vi "Dashboard Main.vi"() -> ()   [LabVIEW 2016]
uses:
  <vilib>/Utility/miscctls.llb/LVRowAndColumnTypeDef.ctl
  <vilib>/event_ctls.llb/eventvkey.ctl
  <vilib>/Rock Robotics/WPI/Dashboard/WPI_DashboardLogging Global.vi
  <vilib>/Rock Robotics/Network Tables/NT Write Boolean.vi
panel:
  in  "Camera Settings Right":T1={"Frame Rate"=15, "Compression"=30, "Size"=1, "DB Camera Config"=FALSE} {"Frame Rate" scale=1.0..30.0; "Compression" scale=100.0..-1.0; "Size" items=["640x480", "320x240", "160x120"]}
  in  "Camera Name Right":string(combo)="No Camera Selection"
  out "Camera Info":cluster{"Mbps LED":bool, "Mbps":dbl, "fps":dbl} {"fps" format="%#.1g"; "Mbps" format="%#.1g"}
  in  "Camera Settings":T1={"Frame Rate"=15, "Compression"=30, "Size"=1, "DB Camera Config"=FALSE} {"Frame Rate" scale=1.0..30.0; "Compression" scale=100.0..-1.0; "Size" items=["640x480", "320x240", "160x120"]}
  in  "TCP":refnum<k5>
  in  "Rec Mode":enum32{"Stop", "Record", "Playback"}(radio)
  out "Robot IP":string
  out "Image Message":string="Timeout in Camera Communications"
  in  "Dashboard Tab":T2(tab)
  out "Pincher State":string
  out "Arm State":string
  in  "Compressor On":bool=TRUE
  in  "Battery Number":string
  in  "Match Number":u32
  out "NT Connection":bool
  out "Gyro":dbl(knob) scale=0.0..360.0
  out "Mode":T3(ring)=enum."Disconnected"
  in  "2 Gear":bool
  in  "Neutral Zone":bool
  in  "Gear Side":enum16{"Center", "Left", "Right"}(ring)
  in  "2 Gear Side":enum16{"Left", "Right"}(ring)
  in  "Alliance":enum16{"Blue", "Red"}(ring)
  in  "Routine":enum16{"Gears", "Nothing", "Reach"}(ring)
  out "Background":bool
  out "Camera Image Right":T4(plugin-control)
  in  "DB/String 9":string
  in  "DB/String 8":string
  in  "DB/String 7":string
  in  "DB/String 6":string
  in  "DB/String 5":string
  in  "DB/String 4":string
  in  "DB/String 3":string
  in  "DB/String 2":string
  in  "DB/String 1":string
  in  "DB/String 0":string
  in  "DB/Slider 0":dbl(slide) scale=0.0..5.0
  in  "DB/Slider 1":dbl(slide) scale=0.0..5.0
  in  "DB/Slider 2":dbl(slide) scale=0.0..5.0
  in  "DB/Slider 3":dbl(slide) scale=0.0..5.0
  out "DB/LED 3":bool
  out "DB/LED 2":bool
  out "DB/LED 1":bool
  out "DB/LED 0":bool
  in  "DB/Button 3":bool
  in  "DB/Button 2":bool
  in  "DB/Button 1":bool
  in  "DB/Button 0":bool caption="New Name"
  in  "Test Slider":dbl(slide) scale=0.0..100.0 scale format="%#_3g"
  in  "On/Off":bool caption="Solenoid"
  in  "Test Name":u16(ring) items=["Select the test to run..."]
  in  "Test Tree":string(tree)
  in  "Motor":cluster{"Value":dbl, "Enable":bool} {"Value" scale=-1.0..1.0 scale format="%#_3g"}
  out "Progress":T5 {"Test Progress" scale=0.0..100.0}
  in  "Rev/Fwd":cluster{"Forward":bool, "Reverse":bool}
  in  "Test Ring":u16(ring) items=["Monochrome", "Color"]
  out "Cmd Status":string
  in  "Execute Command":bool
  in  "Command Params":string[][](table)
  in  "Command Selection":i32(listbox)
  in  "CheckList":i32(listbox)
  out "Tree":string(tree)
  out "Camera Image":T4(plugin-control)
  in  "Camera Name":string(combo)="No Camera Selection"
  # "HW"
  # "HW"
  # "DO NOT PRESS SPACE OR ENTER WHILE ROBOT IS ENABLED!!!"
  # "This tab is a great place for autonomous settings and robot-specific values.\nPlace controls and indicators inside this tab and match name to\nDashboard Variables on robot. You can also delete this comment."
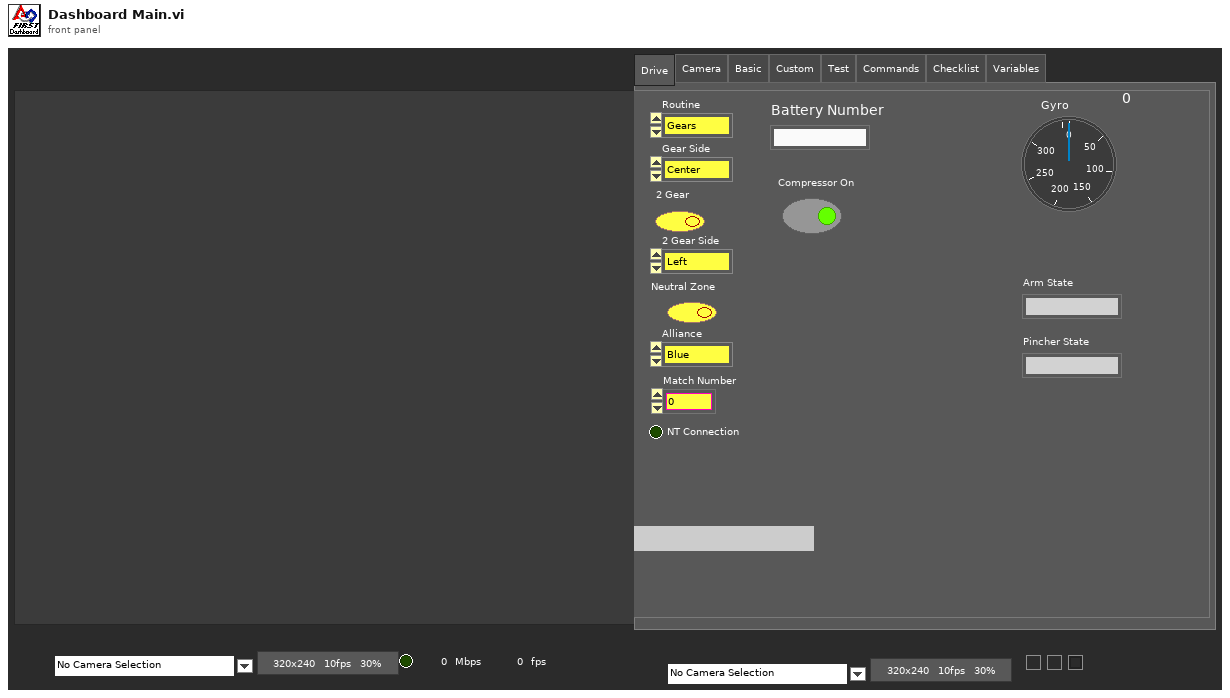
[diagram p1: front panel]
types:
  T1 = cluster{"Frame Rate":i32, "Compression":i32, "Size":u16, "DB Camera Config":bool}
  T2 = enum32{"Drive", "Camera", "Basic", "Custom", "Test", "Commands", "Checklist", "Variables"}
  T3 = enum8{"Tele-Op Disabled", "Tele-Op Enabled", "Auto Disabled", "Auto Enabled", "Test Disabled", "Test Enabled", "Disconnected", "No Code", "E-Stop"}
  T4 = typedef "IMAQ Image.ctl" = refnum<image>
  T5 = cluster{"Test Progress":u8, "Test Progress Text":string}
  T6 = cluster{"IDs":cluster{"RPC field ID":u16, "Unique ID":u16}, "String":string}
  T7 = enum32{"Drive", "Basic", "Custom", "Test", "Checklist", "Variables"}
  T8 = typedef "Image Type" = u32
  T9 = cluster{"Error Strings":string, "Disable Counts":cluster{u16, u16}, "Rail Faults":cluster{u16, u16, u16}, "Robot IP":string, "DB Mode":u8, "Event Info":cluster{"Name":string, "Type":u8, "Number":u16, "Replay":u8}}
  T10 = cluster{"Storage":cluster{"Disk Free":u64, "RAM Block":u32, "RAM free":u32}, "CPU Utilization":cluster{"CPU % ISR":sgl, "CPU % Time Crit":sgl, "CPU % Timed Str":sgl, "CPU % High":sgl, "CPU % Above":sgl, "CPU % Normal":sgl, "CPU % Low":sgl}, "CAN":cluster{"% Bus Utilization":sgl, "Bus Off Cnt":u32, "TX_FIFO Full Cnt":u32, "Receive Error Cnt":u8, "Transmit Error Cnt":u8}, "HID":cluster{"HID Outputs":u32, "Rumble Low":u16, "Rumble High":u16}[]}
  T11 = cluster{"Status bits":cluster{"Test Mode":bool, "Autonomous":bool, "Enabled":bool, "Code Start":bool, "Brownout":bool, "Reserved 2":bool, "Reserved 3":bool, "E-Stop":bool}, "Code Trace":cluster{"Disabled":bool, "TeleOp":bool, "Auto":bool, "Test":bool}, "Controller Type":enum16{"unknown", "cRIO", "roboRio"}, "Code?":enum16{"unknown", "noCode", "code"}, "Battery V":dbl}
  T12 = cluster{"Control Bits":cluster{"TestMode":bool, "Autonomous":bool, "Enabled":bool, "FMS Present":bool, bool, bool, bool, "E-Stop":bool}, "Team Station ":u8, "Countdown":sgl, "Joystick Values":cluster{"Axes":dbl[], "Buttons":bool[], "POVs":i16[]}[]}
  T13 = cluster{"Camera Image":refnum<vi>, "Dashboard Tab":refnum<vi>, "Background":refnum<vi>, "Rec Mode":refnum<vi>, "Test Slider":refnum<vi>, "On/Off ":refnum<vi>, "Test Ring":refnum<vi>, "Rev/Fwd":refnum<vi>, "Test Name":refnum<vi>, "Motor":refnum<vi>, "Progress":refnum<vi>, "CheckList":refnum<vi>, "Tree":refnum<vi>, "Test Tree":refnum<vi>, "Command Params":refnum<vi>, "Command Selection":refnum<vi>, "Execute Command":refnum<vi>, "Cmd Status":refnum<vi>, "Camera Settings":refnum<vi>, "Camera Name":refnum<vi>, "Camera Info":refnum<vi>, "Camera Settings Right":refnum<vi>, "Camera Name Right":refnum<vi>, "Camera Image Right":refnum<vi>}
  T14 = cluster{"Operation":enum16{"Update", "Clear"}, "Color Box":u32}[]
  T15 = typedef "eventvkey.ctl" = enum16{"ASCII", "Enter", "Return", "Shift", "Ctrl", "Alt", "Cmd", "Opt", "Caps", "NumLock", "Clear", "Break", "Up", "Down", "Left", "Right", "Insert", "Delete", "Home", "End", "PageUp", "PageDown", "Escape", "Help", "Pause", "ScrollLock", "F1", "F2", "F3", "F4", "F5", "F6", "F7", "F8", "F9", "F10", "F11", "F12", "F13", "F14", "F15", "F16", "F17", "F18", "F19", "F20", "F21", "F22", "F23", "F24", "Play", "VolumeUp", "VolumeDown", "Mute", "Two Byte Char"}
  T16 = cluster{"Image Size":bool, "Image Type":bool, "Pixel Value":bool, "ROI Information":bool, "Zoom Factor":bool}
  T17 = cluster{"Operation":enum16{"Update", "Clear"}, "Color Box":u32}
  T18 = typedef "LVRowAndColumnTypeDef.ctl" = cluster{"Row":i32, "Column":i32}
  T19 = cluster{"Shift":bool, "Ctrl":bool, "Alt":bool, "Cmd":bool, "Opt":bool}
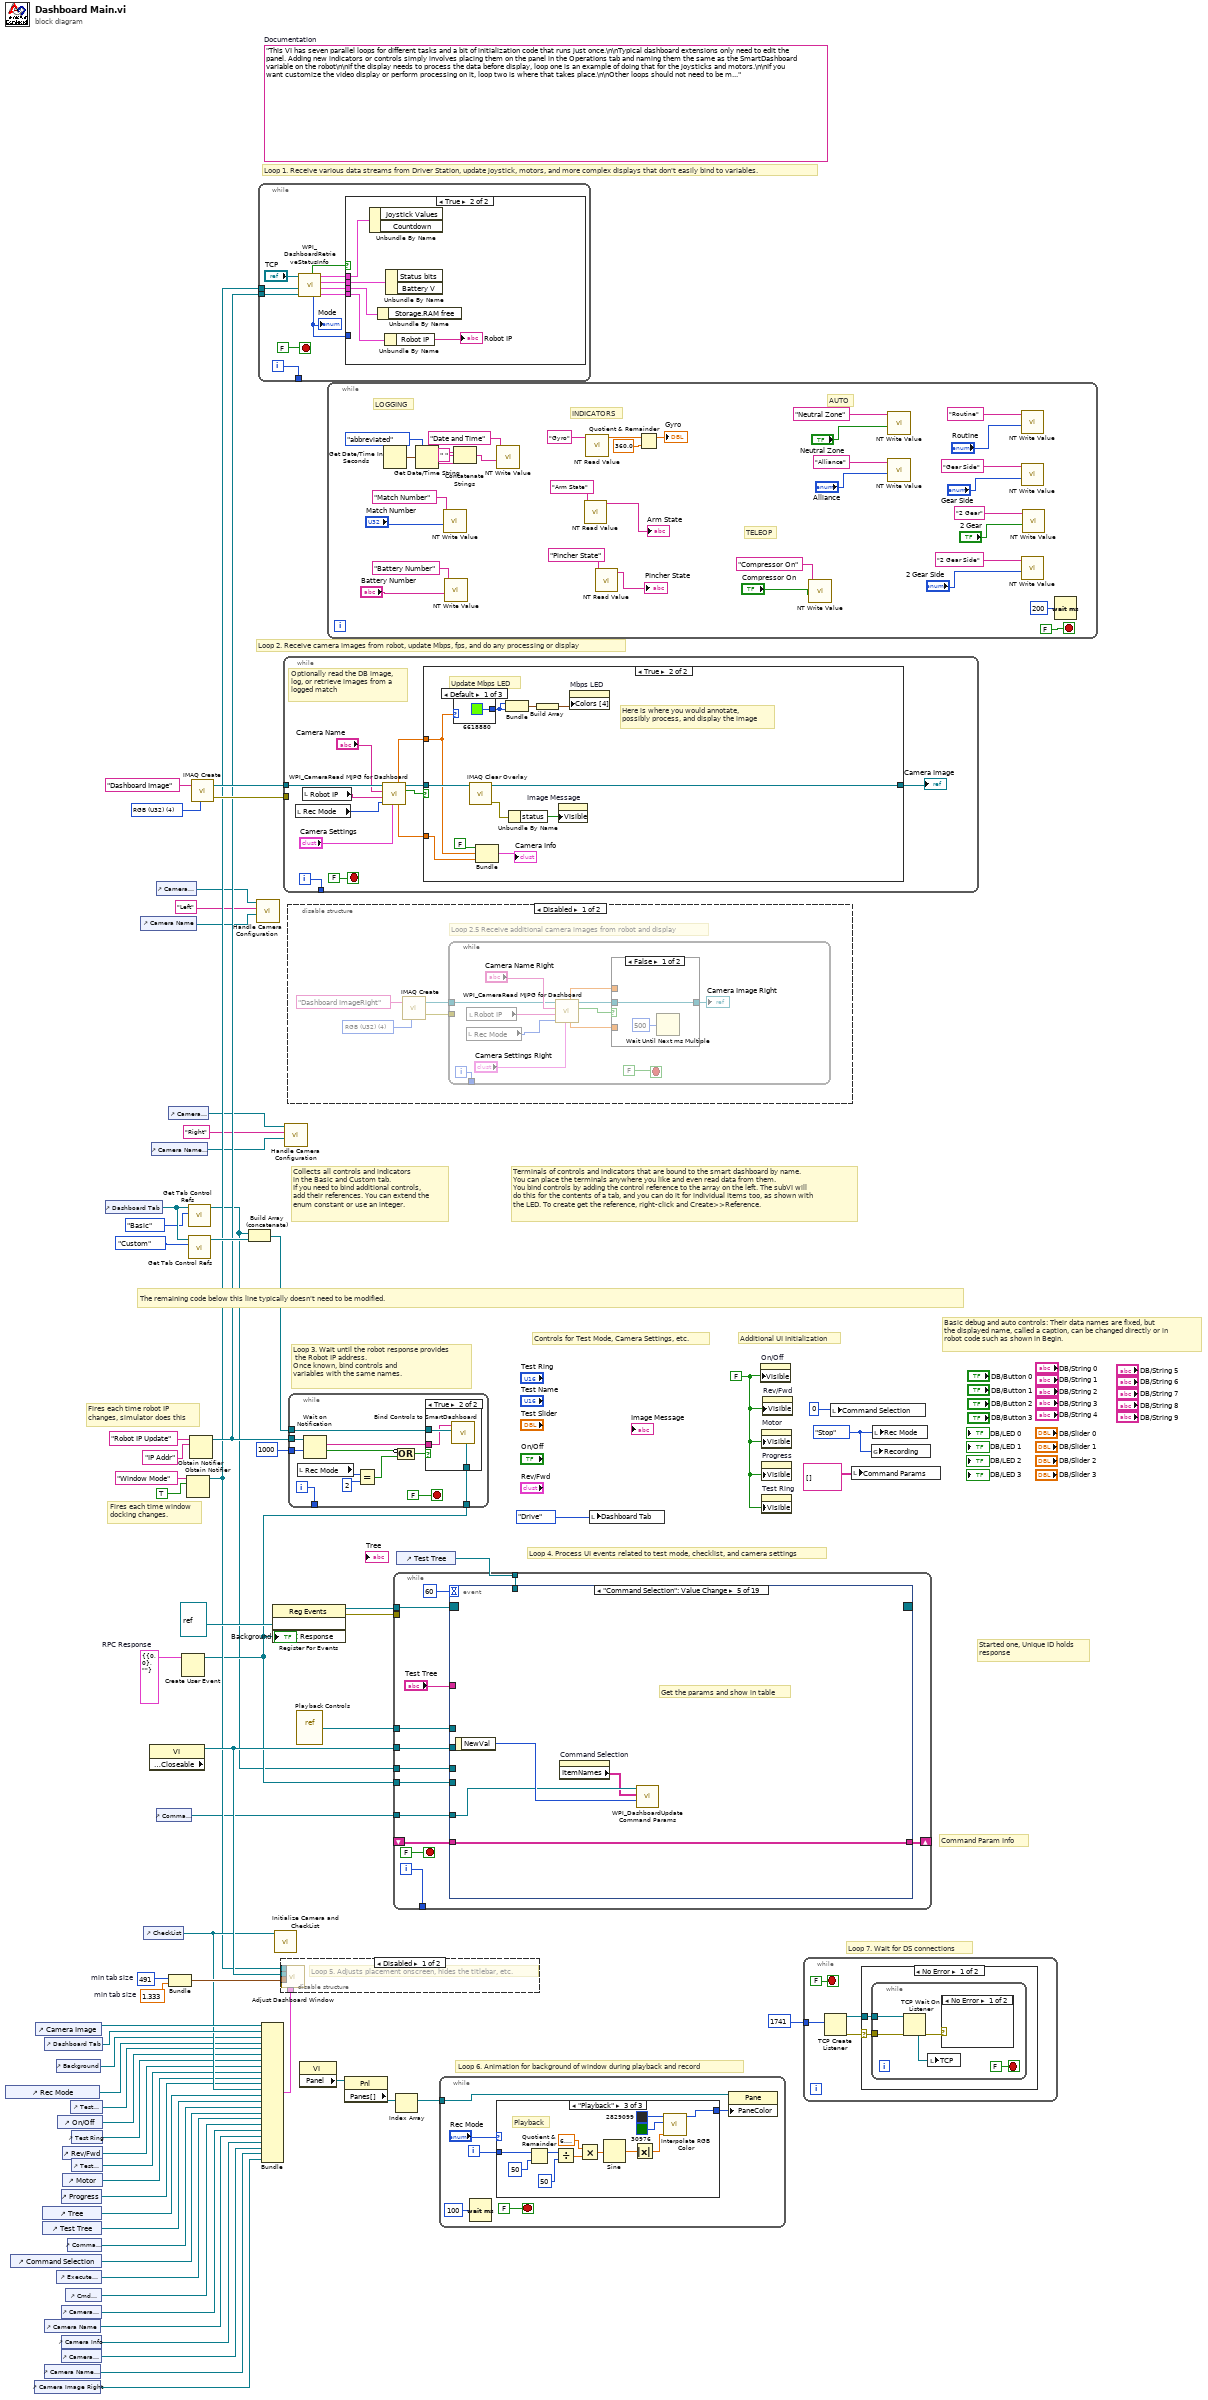
[diagram p0: block diagram]
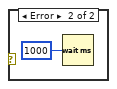
[diagram p5: hidden frame]
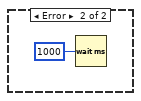
[diagram p6: hidden frame]
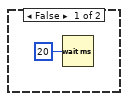
[diagram p7: hidden frame]
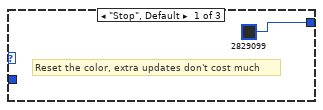
[diagram p8: hidden frame]
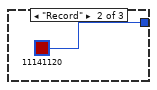
[diagram p9: hidden frame]
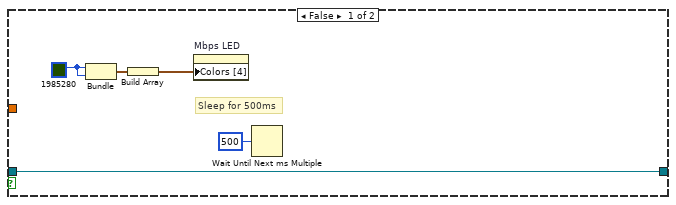
[diagram p11: hidden frame]
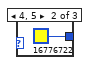
[diagram p12: hidden frame]
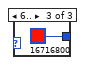
[diagram p13: hidden frame]
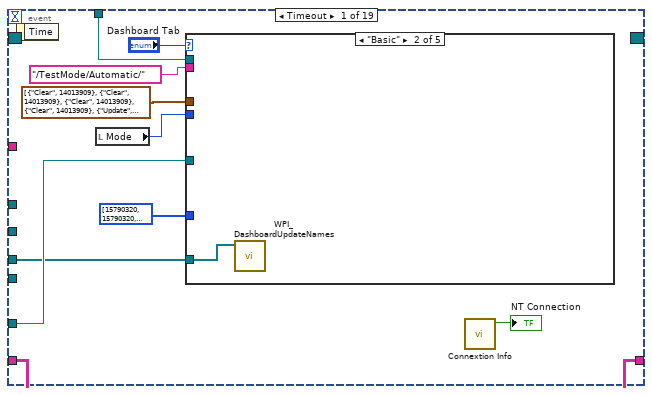
[diagram p14: hidden frame]
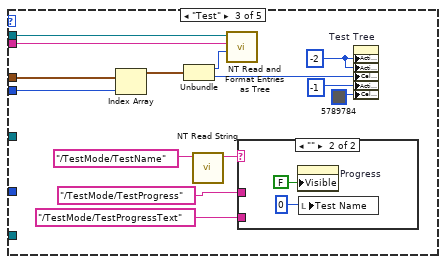
[diagram p16: hidden frame]
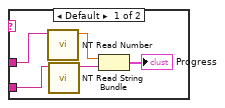
[diagram p17: hidden frame]
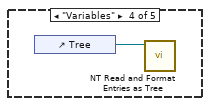
[diagram p18: hidden frame]
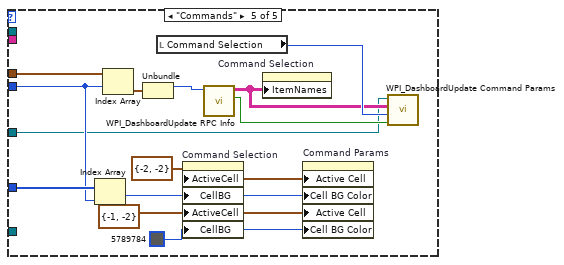
[diagram p19: hidden frame]
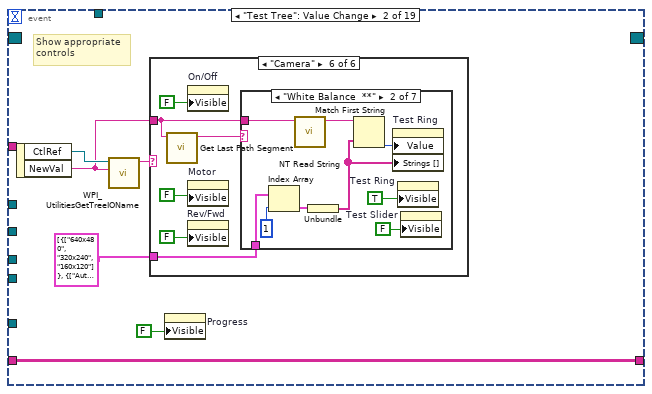
[diagram p20: hidden frame]
diagram:
  w22 = T6 {"IDs"={"RPC field ID"=0, "Unique ID"=0}, "String"=""}  # RPC Response
  w45 = 491  # min tab size
  w44 = 1.333  # min tab size
  w52 = enum32{"Stop", "Record", "Playback"}."Stop" ("Rec Mode")
  w29 = FALSE ("Visible")
  (unwired) "This VI has seven parallel loops for different tasks and a bit of initialization code that runs just once.\n\nTypical dashboard extensions only need to edit the panel. Adding new indicators or controls simply involves placing them on the panel in the Operations tab and naming them the same as the SmartDashboard variable on the robot\n\nIf the display needs to process the data before display, loop one is an example of doing that for the joysticks and motors.\n\nIf you want customize the video display or perform processing on it, loop two is where that takes place.\n\nOther loops should not need to be modified. They are pretty standard, and document the task they perform."  # Documentation
  w69 = T8 4 items=["Grayscale (U8)", "Grayscale (I16)", "Grayscale (SGL)", "Complex (CSG)", "RGB (U32)", "HSL (U32)", "RGB (U64)"] ("Image Type")
  # "Command Param Info"
  # "Started one, Unique ID holds\nresponse"
  # "Loop 7. Wait for DS connections"
  # "Basic debug and auto controls: Their data names are fixed, but\nthe displayed name, called a caption, can be changed directly or in\nrobot code such as shown in Begin."
  # "Controls for Test Mode, Camera Settings, etc."
  # "Additional UI Initialization"
  # "Loop 6. Animation for background of window during playback and record"
  # "Fires each time robot IP\nchanges, simulator does this"
  # "Fires each time window\ndocking changes."
  # "Collects all controls and indicators\nin the Basic and Custom tab.\nIf you need to bind additional controls,\nadd their references. You can extend the\nenum constant or use an integer."
  # "The remaining code below this line typically doesn't need to be modified."
  # "Loop 4. Process UI events related to test mode, checklist, and camera settings"
  # "Terminals of controls and indicators that are bound to the smart dashboard by name.\nYou can place the terminals anywhere you like and even read data from them.\nYou bind controls by adding the control reference to the array on the left. The subVI will\ndo this for the contents of a tab, and you can do it for individual items too, as shown with\nthe LED. To create get the reference, right-click and Create>>Reference."
  # "Loop 3. Wait until the robot response provides\n the Robot IP address.\nOnce known, bind controls and\nvariables with the same names."
  # "Loop 1. Receive various data streams from Driver Station, update joystick, motors, and more complex displays that don't easily bind to variables."
  # "Loop 2. Receive camera images from robot, update Mbps, fps, and do any processing or display"
  n1 = control-ref of="Rec Mode"() -> (w35:refnum<vi>)
  n2 = control-ref of="Command Selection"() -> (w21:refnum<vi>)
  n3 = control-ref of="Camera Image Right"() -> (w3:refnum<vi>)
  n4 = control-ref of="Camera Image"() -> (w47:refnum<vi>)
  n5 = control-ref of="Tree"() -> (w39:refnum<vi>)
  n6 = control-ref of="Test Tree"() -> (w38:refnum<vi>)
  n7 = control-ref of="Dashboard Tab"() -> (w46:refnum<vi>)
  n8 = control-ref of="Camera Name"() -> (w12:refnum<vi>)
  n9 = control-ref of="Camera Name Right"() -> (w4:refnum<vi>)
  n10 = control-ref of="Background"() -> (w2:refnum<vi>)
  n11 = control-ref of="Execute Command"() -> (w23:refnum<vi>)
  n12 = control-ref of="On/Off"() -> (w33:refnum<vi>)
  n13 = control-ref of="Progress"() -> (w30:refnum<vi>)
  n14 = control-ref of="Camera Settings"() -> (w13:refnum<vi>)
  n15 = control-ref of="Camera Info"() -> (w11:refnum<vi>)
  n16 = control-ref of="Camera Settings Right"() -> (w5:refnum<vi>)
  n17 = control-ref of="Rev/Fwd"() -> (w31:refnum<vi>)
  n18 = control-ref of="Motor"() -> (w36:refnum<vi>)
  n19 = control-ref of="Cmd Status"() -> (w17:refnum<vi>)
  n20 = control-ref of="Command Params"() -> (w24:refnum<vi>)
  n21 = control-ref of="Test Slider"() -> (w34:refnum<vi>)
  n22 = control-ref of="Test Ring"() -> (w32:refnum<vi>)
  n23 = control-ref of="Test Name"() -> (w37:refnum<vi>)
  n24 = control-ref of="Dashboard Tab"() -> (w50:refnum<vi>)
  n25 = control-ref of="Camera Name"() -> (w14:refnum<vi>)
  n26 = control-ref of="CheckList"() -> (w40:refnum<vi>)
  n27 = property class="VI" props=["Front Panel.Closeable"]() -> (reference out=w51:refnum<vi>)  [unwired: 2 in, 2 out]
  n28 = control-ref of="Camera Name Right"() -> (w8:refnum<vi>)
  n29 = control-ref of="Camera Settings"() -> (w15:refnum<vi>)
  n30 = control-ref of="Command Params"() -> (w16:refnum<vi>)
  n31 = control-ref of="Camera Settings Right"() -> (w9:refnum<vi>)
  n32 = Bundle("min tab size"=w45, "min tab size"=w44) -> (w43:cluster{"min tab size":i32, "min tab size":dbl})  [unwired: 1 in]
  n33 = Create User Event(user event datatype=w22) -> (user event=w18:refnum<user-event>)  [unwired: 1 in, 1 out]
  n34 = Obtain Notifier(name (unnamed)="Window Mode", notification data type=TRUE) -> (notifier out=w27:refnum<notifier>)  [unwired: 2 in, 2 out]
  n35 = call <vilib>:"Get Tab Control Refs.vi"("Page Index"=T7."Basic" ("Dashboard Tab"), "TabControl in"=w50) -> ("ControlsOnPage"=w10:refnum<vi>[])  [unwired: 9 in]
  n36 = call <vilib>:"Get Tab Control Refs.vi"("Page Index"=T7."Custom" ("Dashboard Tab"), "TabControl in"=w50) -> ("ControlsOnPage"=w49:refnum<vi>[])  [unwired: 9 in]
  n37 = Obtain Notifier(name (unnamed)="Robot IP Update", notification data type="IP Addr" ("name (unnamed)")) -> (notifier out=w28:refnum<notifier>)  [unwired: 2 in, 2 out]
  n38 = call "IMAQ Create"("Image Name"="Dashboard Image", "Image Type"=w69) -> ("New Image"=w67:T4, "error out"=w66:errorcluster)  [unwired: 2 in, 1 out]
  n39 = Build Array (concatenate)(w10, w49) -> (w48:refnum<vi>[])
  n40 = call "Handle Camera Configuration.vi"("CameraNameRef"=w14, "Camera File Name"="Left", "ClusterRef"=w15) -> ()  [unwired: 9 in]
  n41 = while {
    tunnel: w28 -> [w74]
    tunnel: w27 -> [w71]
    tunnel: [w70] -> _
    i -> [w70]
    stop <- FALSE stop-if-true
    n42 = call <vilib>:"WPI_DashboardRetrieveStatusInfo.vi"("Binding Refnum"=w74, "Window Mode Notifier"=w71, "TCP Cnx"="TCP") -> ("Power and Errors"=w75:T9, "Robot Metrics"=w78:T10, "Status Info"=w79:T11, "Control Info"=w76:T12, "Robot Mode"=w73:T3, "Process?"=w77:bool)  [unwired: 3 in]
    "Mode" <- w73
    n43 = case shown="True" w77 {
      tunnel: w79 -> [_ w86]
      tunnel: w78 -> [_ w85]
      tunnel: w76 -> [_ w84]
      tunnel: w75 -> [_ w83]
      tunnel: w73 -> [_ _]
      frame False {
        n44 = Wait (ms)(milliseconds to wait=u32 20) -> ()  [unwired: 1 out]
      }
      frame True {
        n45 = Unbundle By Name(w84) -> ()  [unwired: 2 out]
        n46 = Unbundle By Name(w85) -> ()  [unwired: 1 out]
        n47 = Unbundle By Name(w83) -> ("Robot IP"=→"Robot IP":string)
        n48 = Unbundle By Name(w86) -> ()  [unwired: 2 out]
      }
    }
  }
  n49 = Bundle("Camera Image"=w47, "Dashboard Tab"=w46, "Background"=w2, "Rec Mode"=w35, "Test Slider"=w34, "On/Off"=w33, "Test Ring"=w32, "Rev/Fwd"=w31, "Test Name"=w37, "Motor"=w36, "Progress"=w30, "CheckList"=w40, "Tree"=w39, "Test Tree"=w38, "Command Params"=w24, "Command Selection"=w21, "Execute Command"=w23, "Cmd Status"=w17, "Camera Settings"=w13, "Camera Name"=w12, "Camera Info"=w11, "Camera Settings Right"=w5, "Camera Name Right"=w4, "Camera Image Right"=w3) -> (w1:T13)  [unwired: 1 in]
  n50 = register-events(refnum<vi> refnum, w18) -> (reference out=w56:refnum<event-registration>, error out=w55:errorcluster)  [unwired: 2 in]
  n51 = call "Initialize Camera and CheckList.vi"("ListBox in"=w40) -> ()  [unwired: 11 in]
  n52 = disable-structure shown="Disabled" {
    disable-tunnel: w51 -> [w90 _]
    disable-tunnel: w43 -> [w89 _]
    disable-tunnel: w27 -> [w88 _]
    disable-tunnel: w1 -> [w87 _]
    frame Disabled {
      # "Loop 5. Adjusts placement onscreen, hides the titlebar, etc."
      n53 = call "Adjust Dashboard Window.vi"("Sizing Refnums"=w87, "Size Constraints"=w89, "VI"=w90, "WIn Mode"=w88) -> ()  [unwired: 8 in]
    }
    frame Enabled {
    }
  }
  n54 = while {
    tunnel: w67 -> [w100]
    tunnel: w66 -> [_]
    tunnel: [w101] -> _
    i -> [w101]
    stop <- FALSE stop-if-true
    # "Optionally read the DB image,\nlog, or retrieve images from a\nlogged match"
    n55 = local read "Rec Mode"() -> (w96:enum32{"Stop", "Record", "Playback"})
    n56 = local read "Robot IP"() -> (w95:string)
    n57 = call <vilib>:"WPI_CameraRead MJPG for Dashboard.vi"("Camera Settings"="Camera Settings", "Rec Mode"=w96, "Robot IP"=w95, "Camera Name"="Camera Name", "Refnum in"=w100) -> ("Active"=w98:bool, "Refnum out"=w99:T4, "FPS"=w97:dbl, "Bandwidth (Mbps)"=w94:dbl)  [unwired: 3 in]
    n58 = case shown="True" w98 {
      tunnel: w99 -> [w103 w114]
      tunnel: w94 -> [_ w111]
      tunnel: w97 -> [_ w112]
      tunnel: [w103 w108] -> w91
      frame False {
        w105 = u32 1985280 ("Color Box")
        # "Sleep for 500ms"
        n59 = Bundle("Color Box"=w105, "Color Box"=w105) -> (w106:cluster{"Color Box":u32, "Color Box":u32})  [unwired: 1 out]
        n60 = Build Array(w106) -> (w104:cluster{"Color Box":u32, "Color Box":u32}[])
        n61 = property on="Mbps LED" class="Bool (strict)"("Colors [4]"=w104) -> ()  [unwired: 2 in, 2 out]
        n62 = Wait Until Next ms Multiple(millisecond multiple=u32 500) -> ()  [unwired: 1 out]
      }
      frame True {
        # "Here is where you would annotate,\npossibly process, and display the image"
        # "Update Mbps LED"
        n63 = case shown="Default" w111 {
          tunnel: [u32 6618880 ("Color Box") u32 16776722 ("Color Box") u32 16716800 ("Color Box")] -> w115
          frame Default {
          }
          frame 4, 5 {
          }
          frame 6.. {
          }
        }
        n64 = call "IMAQ Clear Overlay"("Image"=w114) -> ("error out"=w117:errorcluster, "Image Out"=w108:T4)  [unwired: 2 in, 7 out]
        n65 = Bundle(FALSE, "Bandwidth (Mbps)"=w111, "FPS"=w112) -> (→"Camera Info":cluster{bool, "Bandwidth (Mbps)":dbl, "FPS":dbl})  [unwired: 1 in]
        n66 = Bundle("Color Box"=w115, "Color Box"=w115) -> (w116:cluster{"Color Box":u32, "Color Box":u32})  [unwired: 1 out]
        n67 = Unbundle By Name(w117) -> ("status"=w118:bool)
        n68 = Build Array(w116) -> (w113:cluster{"Color Box":u32, "Color Box":u32}[])
        n69 = property on="Image Message" class="Str"("Visible"=w118) -> ()  [unwired: 2 in, 2 out]
        n70 = property on="Mbps LED" class="Bool (strict)"("Colors [4]"=w113) -> ()  [unwired: 2 in, 2 out]
      }
    }
    "Camera Image" <- w91
  }
  n71 = call "Handle Camera Configuration.vi"("CameraNameRef"=w8, "Camera File Name"="Right", "ClusterRef"=w9) -> ()  [unwired: 9 in]
  n72 = disable-structure shown="Disabled" {
    frame Disabled {
      w124 = T8 4 items=["Grayscale (U8)", "Grayscale (I16)", "Grayscale (SGL)", "Complex (CSG)", "RGB (U32)", "HSL (U32)", "RGB (U64)"] ("Image Type")
      # "Loop 2.5 Receive additional camera images from robot and display"
      n73 = call "IMAQ Create"("Image Name"="Dashboard ImageRight", "Image Type"=w124) -> ("New Image"=w123:T4, "error out"=w122:errorcluster)  [unwired: 2 in, 1 out]
      n74 = while {
        tunnel: w123 -> [w136]
        tunnel: w122 -> [_]
        tunnel: [w130] -> _
        i -> [w130]
        stop <- FALSE stop-if-true
        n75 = local read "Rec Mode"() -> (w134:enum32{"Stop", "Record", "Playback"})
        n76 = local read "Robot IP"() -> (w135:string)
        n77 = call <vilib>:"WPI_CameraRead MJPG for Dashboard.vi"("Camera Settings"="Camera Settings Right", "Rec Mode"=w134, "Robot IP"=w135, "Camera Name"="Camera Name Right", "Refnum in"=w136) -> ("Active"=w129:bool, "Refnum out"=w132:T4, "FPS"=w127:dbl, "Bandwidth (Mbps)"=w128:dbl)  [unwired: 3 in]
        n78 = case shown="False" w129 {
          tunnel: w132 -> [w138 w140]
          tunnel: w128 -> [_ _]
          tunnel: w127 -> [_ _]
          tunnel: [w138 w140] -> w126
          frame False {
            n79 = Wait Until Next ms Multiple(millisecond multiple=u32 500) -> ()  [unwired: 1 out]
          }
          frame True {
          }
        }
        "Camera Image Right" <- w126
      }
    }
    frame Enabled {
    }
  }
  n80 = while {
    tunnel: w48 -> [w152]
    tunnel: w28 -> [w150]
    tunnel: [w148] -> _
    tunnel: u32 1000 ("milliseconds to wait") -> [w147]
    tunnel: w18 -> [w141]
    i -> [w148]
    stop <- FALSE stop-if-true
    n81 = local read "Rec Mode"() -> (w143:enum32{"Stop", "Record", "Playback"})
    n82 = Wait on Notification(notifier=w150, timeout in ms (-1)=w147) -> (notification=w149:string, timed out?=w145:bool)  [unwired: 2 in, 2 out]
    n83 = Equal?(x=w143, y=u16 2 ("Rec Mode")) -> (x = y?=w144:bool)
    n84 = Compound Arithmetic op=OR(invert w145, w144) -> (w146:bool)
    n85 = case shown="True" w146 {
      tunnel: w152 -> [_ w155]
      tunnel: w149 -> [_ w154]
      tunnel: w141 -> [_ w153]
      frame False {
      }
      frame True {
        n86 = call <vilib>:"Bind Controls to SmartDashboard.vi"("RPC ref"=w153, "Bound Control Refs"=w155, "Server IP Address"=w154) -> ()  [unwired: 9 in]
      }
    }
  }
  n87 = vi-ref "Playback Controls.vi"() -> (w57:refnum<vi>)
  n88 = property class="VI"() -> ("Panel"=w59:refnum<vi>)  [unwired: 2 in, 2 out]
  n89 = while {
    stop <- FALSE stop-if-true
    # "TELEOP"
    # "AUTO"
    # "INDICATORS"
    # "LOGGING"
    n90 = Get Date/Time In Seconds() -> (seconds since 1Jan1904=w188:timestamp)
    n91 = Get Date/Time String(date format (0)=enum16{"short", "long", "abbreviated"}."abbreviated", seconds (now)=w188) -> (date string=w185:string, time string=w186:string)  [unwired: 1 in]
    n92 = call-poly <vilib>:"NT Write Value.vi"("Numeric"="Match Number", "Name"="Match Number") -> ()  [unwired: 9 in, 1 out]
    n93 = call-poly <vilib>:"NT Write Value.vi"("String"="Battery Number", "Name"="Battery Number") -> ()  [unwired: 9 in, 1 out]
    n94 = Concatenate Strings(w185, " " ("string"), w186) -> (w168:string)
    n95 = call-poly <vilib>:"NT Write Value.vi"("String"=w168, "Name"="Date and Time") -> ()  [unwired: 9 in, 1 out]
    n96 = call-poly <vilib>:"NT Read Value.vi"("Name"="Arm State") -> ("String"=→"Arm State":string)  [unwired: 9 in, 1 out]
    n97 = call-poly <vilib>:"NT Read Value.vi"("Name"="Gyro") -> ("Numeric"=w166:dbl)  [unwired: 9 in, 1 out]
    n98 = call-poly <vilib>:"NT Read Value.vi"("Name"="Pincher State") -> ("String"=→"Pincher State":string)  [unwired: 9 in, 1 out]
    n99 = Quotient & Remainder(x=w166, y=360.0) -> (x-y*floor(x/y)=→"Gyro":dbl)  [unwired: 1 out]
    n100 = call-poly <vilib>:"NT Write Value.vi"("Boolean"="Compressor On", "Name"="Compressor On") -> ()  [unwired: 9 in, 1 out]
    n101 = call-poly <vilib>:"NT Write Value.vi"("Boolean"="Neutral Zone", "Name"="Neutral Zone") -> ()  [unwired: 9 in, 1 out]
    n102 = call-poly <vilib>:"NT Write Value.vi"("Numeric"="Alliance", "Name"="Alliance") -> ()  [unwired: 9 in, 1 out]
    n103 = call-poly <vilib>:"NT Write Value.vi"("Numeric"="Routine", "Name"="Routine") -> ()  [unwired: 9 in, 1 out]
    n104 = call-poly <vilib>:"NT Write Value.vi"("Numeric"="Gear Side", "Name"="Gear Side") -> ()  [unwired: 9 in, 1 out]
    n105 = call-poly <vilib>:"NT Write Value.vi"("Numeric"="2 Gear Side", "Name"="2 Gear Side") -> ()  [unwired: 9 in, 1 out]
    n106 = call-poly <vilib>:"NT Write Value.vi"("Boolean"="2 Gear", "Name"="2 Gear") -> ()  [unwired: 9 in, 1 out]
    n107 = Wait (ms)(milliseconds to wait=u32 200) -> ()  [unwired: 1 out]
  }
  n108 = property class="Pnl"(reference=w59) -> ("Panes[]"=w60:refnum<vi>[])  [unwired: 1 in, 2 out]
  n109 = Index Array(array=w60) -> (element=w58:refnum<vi>)  [unwired: 1 in]
  n110 = control-ref of="Test Tree"() -> (w61:refnum<vi>)
  n111 = while {
    tunnel: [w200] -> _
    tunnel: w61 -> [w199]
    tunnel: w57 -> [w198]
    tunnel: w56 -> [w197]
    tunnel: w55 -> [_]
    tunnel: w51 -> [w196]
    tunnel: w18 -> [w195]
    tunnel: w16 -> [w194]
    shift-right: [w193] -> _
    shift-left: _ -> [w192]
    tunnel: w10 -> [w191]
    i -> [w200]
    stop <- FALSE stop-if-true
    n112 = event shown="[4] \"Command Selection\": Value Change" {
      selector: w197 -> [_ _ _ _ _ _ _ _ _ _ _ _ _ _ _ _ _ _ _]
      dyn-events: [_ _ _ _ _ _ _ _ _ _ _ _ _ _ w450 _ _ _ _] -> _
      timeout: u32 60 ("milliseconds to wait") -> [_ _ _ _ _ _ _ _ _ _ _ _ _ _ _ _ _ _ _]
      tunnel: w199 -> [w212 _ _ _ _ _ _ _ _ _ _ _ _ _ _ _ _ _ _]
      tunnel: "Test Tree" -> [_ _ _ _ _ _ _ _ _ w417 w425 w427 w431 w439 _ _ _ _ _]
      tunnel: w198 -> [_ _ _ _ _ _ _ _ _ _ _ _ _ _ w452 _ w470 _ _]
      tunnel: w196 -> [_ _ _ _ _ _ _ _ _ _ _ _ _ _ w448 _ _ _ _]
      tunnel: w195 -> [_ _ _ _ _ _ _ _ _ _ _ _ _ _ w444 _ _ _ _]
      tunnel: w194 -> [w207 _ _ _ w368 _ _ _ _ _ _ _ _ _ _ _ _ _ _]
      tunnel: [w206 w251 w353 w358 w366 w375 w385 w392 w404 w416 w423 w426 w430 w438 w443 w465 w467 w471 w482] -> w193
      tunnel: w192 -> [w206 w251 w353 w358 w366 _ _ w392 w404 w416 w423 w426 w430 w438 w443 w465 w467 w471 w482]
      tunnel: w191 -> [w204 _ _ _ _ _ _ _ _ _ _ _ _ _ _ _ _ _ _]
      event Timeout {
        n113 = event-data() -> ()  [unwired: 1 in, 1 out]
        n114 = local read "Mode"() -> (w209:T3)
        n115 = case shown="\"Basic\"" "Dashboard Tab" {
          tunnel: w212 -> [_ _ w228 _ _]
          tunnel: "/TestMode/Automatic/" ("Name Pattern") -> [_ _ w227 _ _]
          tunnel: T14 [{"Operation"=enum."Clear", "Color Box"=14013909}, {"Operation"=enum."Clear", "Color Box"=14013909}, {"Operation"=enum."Clear", "Color Box"=14013909}, {"Operation"=enum."Clear", "Color Box"=14013909}, {"Operation"=enum."Update", "Color Box"=14013909}, {"Operation"=enum."Update", "Color Box"=16777215}, {"Operation"=enum."Clear", "Color Box"=14013909}, {"Operation"=enum."Clear", "Color Box"=14013909}, {"Operation"=enum."Clear", "Color Box"=14013909}] -> [_ _ w220 _ w244]
          tunnel: w209 -> [_ _ w219 _ w243]
          tunnel: u32[] [15790320, 15790320, 15790320, 15790320, 16777215, 16777215, 15790320, 15790320, 15790320] -> [_ _ _ _ w249]
          tunnel: w207 -> [_ _ _ _ w237]
          tunnel: w204 -> [_ w214 _ _ _]
          frame "Custom", Default {
          }
          frame "Basic" {
            n116 = call <vilib>:"WPI_DashboardUpdateNames.vi"("Controls on Tab"=w214) -> ()  [unwired: 11 in]
          }
          frame "Test" {
            w226 = -2 ("Active Item:Row Number")
            n117 = Index Array(array=w220, index=w219) -> (element=w221:T17)
            n118 = Unbundle(w221) -> ("Operation"=w222:enum16{"Update", "Clear"}, "Color Box"=w223:u32)
            n119 = call <vilib>:"NT Read String.vi"("Name"="/TestMode/TestName") -> ("String"=w217:string)  [unwired: 9 in, 1 out]
            n120 = call <vilib>:"NT Read and Format Entries as Tree.vi"("Operation"=w222, "Name Pattern"=w227, "Tree Refnum"=w228) -> ()  [unwired: 7 in, 2 out]
            n121 = case shown="\"\"" w217 {
              tunnel: "/TestMode/TestProgress" ("Name") -> [w230 _]
              tunnel: "/TestMode/TestProgressText" ("Name") -> [w229 _]
              frame Default {
                n122 = call <vilib>:"NT Read Number.vi"("Name"=w230) -> ("Numeric"=w231:dbl)  [unwired: 9 in, 1 out]
                n123 = call <vilib>:"NT Read String.vi"("Name"=w229) -> ("String"=w232:string)  [unwired: 9 in, 1 out]
                n124 = Bundle("Numeric"=w231, "String"=w232) -> (→"Progress":cluster{"Numeric":dbl, "String":string})  [unwired: 1 in]
              }
              frame "" {
                n125 = property on="Progress" class="Clust (strict)"("Visible"=FALSE) -> ()  [unwired: 2 in, 2 out]
                n126 = local write "Test Name"(u16 0) -> ()
              }
            }
            n127 = property on="Test Tree" class="Tree (strict)"("Active Item Row Number"=w226, "ActiveColNum"=w226, "CellBG"=w223, "Active Item Row Number"=-1 ("Active Item:Row Number"), "CellBG"=u32 5789784 ("Color Box")) -> ()  [unwired: 2 in, 2 out]
          }
          frame "Variables" {
            n128 = control-ref of="Tree"() -> (w236:refnum<vi>)
            n129 = call <vilib>:"NT Read and Format Entries as Tree.vi"("Tree Refnum"=w236) -> ()  [unwired: 9 in, 2 out]
          }
          frame "Commands" {
            w245 = u32 5789784 ("Color Box")
            w246 = T18 {"Row"=-1, "Column"=-2} ("Active Cell:Active Cell")
            w248 = T18 {"Row"=-2, "Column"=-2} ("Active Cell:Active Cell")
            n130 = Index Array(array=w249, index=w243) -> (element=w247:u32)
            n131 = Index Array(array=w244, index=w243) -> (element=w242:T17)
            n132 = Unbundle(w242) -> ("Operation"=w241:enum16{"Update", "Clear"})  [unwired: 1 out]
            n133 = local read "Command Selection"() -> (w240:i32)
            n134 = property on="Command Selection" class="MCListbox (strict)"("ActiveCell"=w248, "CellBG"=w247, "ActiveCell"=w246, "CellBG"=w245) -> ()  [unwired: 2 in, 2 out]
            n135 = call <vilib>:"WPI_DashboardUpdate RPC Info.vi"("Operation"=w241) -> ("update"=w239:bool, "commands"=w238:string[][])  [unwired: 9 in]
            n136 = property on="Command Selection" class="MCListbox (strict)"("ItemNames"=w238) -> ()  [unwired: 2 in, 2 out]
            n137 = property on="Command Params" class="Tbl (strict)"("Active Cell"=w248, "Cell BG Color"=w247, "Active Cell"=w246, "Cell BG Color"=w245) -> ()  [unwired: 2 in, 2 out]
            n138 = call <vilib>:"WPI_DashboardUpdate Command Params.vi"("Update"=w239, "NewVal"=w240, "Commands"=w238, "Param Tbl"=w237) -> ()  [unwired: 7 in, 1 out]
          }
        }
        n139 = call <vilib>:"Connextion Info.vi"() -> ("Connected"=→"NT Connection":bool)  [unwired: 10 in, 1 out]
      }
      event "Test Tree": Value Change {
        # "Show appropriate\ncontrols"
        n140 = event-data() -> ("CtlRef"=w254:refnum<vi>, "NewVal"=w252:string)  [unwired: 1 in]
        n141 = call <vilib>:"WPI_UtilitiesGetTreeIOName.vi"("NewVal"=w252, "TreeControl in"=w254) -> ("I/O Name"=w255:string)  [unwired: 9 in]
        n142 = case shown="\"Camera\"" w255 {
          selector: w255 -> [_ w262 _ w284 w293 _]
          tunnel: w252 -> [_ _ w281 w283 _ w300]
          tunnel: cluster{string[]}[] [{["640x480", "320x240", "160x120"]}, {["Auto", "Fixed indoor", "Fixed outdoor 1", "Fixed outdoor 2", "Fixed fluorescent 1", "Fixed fluorescent 2", "Hold current"]}, {["Auto", "Flicker-free 50 Hz", "Flicker-free 60 Hz", "Hold current"]}, {["None", "Prioritize frame rate", "Prioritize image quality"]}, {["Monochrome", "Color"]}] -> [_ _ _ _ _ w299]
          frame Default {
            w257 = FALSE ("Visible")
            w256 = FALSE ("Visible")
            n143 = property on="Motor" class="Clust (strict)"("Visible"=w256) -> ()  [unwired: 2 in, 2 out]
            n144 = property on="Test Ring" class="Ring (strict)"("Visible"=w256) -> ()  [unwired: 2 in, 2 out]
            n145 = property on="Rev/Fwd" class="Clust (strict)"("Visible"=w257) -> ()  [unwired: 2 in, 2 out]
            n146 = property on="On/Off" class="Bool (strict)"("Visible"=w257) -> ()  [unwired: 2 in, 2 out]
            n147 = property on="Test Slider" class="Slide (strict)"("Visible"=w257) -> ()  [unwired: 2 in, 2 out]
          }
          frame "Analog Out", "Motor", "PWM" {
            w263 = FALSE ("Visible")
            n148 = case shown="\"Analog Out\"" w262 {
              tunnel: [1.0 ("Value") -1.0 ("Value") 0.0 ("Value")] -> w261
              tunnel: [255.0 ("Value") 1.0 ("Value") 5.0 ("Value")] -> w260
              tunnel: [128.0 ("Value") 0.0 ("Value") 0.0 ("Value")] -> w259
              tunnel: [64.0 ("Value") 0.5 ("Value") 1.0 ("Value")] -> w258
              frame "PWM" {
              }
              frame "Motor", Default {
              }
              frame "Analog Out" {
              }
            }
            n149 = property on="Motor" class="Clust (strict)"("Visible"=TRUE) -> ()  [unwired: 2 in, 2 out]
            n150 = property on="Value" class="Slide (strict)"("Value"=w259, "Scale.Minimum"=w261, "Scale.Maximum"=w260, "Scale.Increment"=w258) -> ()  [unwired: 2 in, 2 out]
            n151 = property on="On/Off" class="Bool (strict)"("Visible"=w263) -> ()  [unwired: 2 in, 2 out]
            n152 = property on="Test Slider" class="Slide (strict)"("Visible"=w263) -> ()  [unwired: 2 in, 2 out]
            n153 = property on="Test Ring" class="Ring (strict)"("Visible"=w263) -> ()  [unwired: 2 in, 2 out]
            n154 = property on="Rev/Fwd" class="Clust (strict)"("Visible"=w263) -> ()  [unwired: 2 in, 2 out]
          }
          frame "Servo" {
            w279 = FALSE ("Visible")
            n155 = call <vilib>:"NT Read Number.vi"("Name"=w281) -> ("Numeric"=w280:dbl)  [unwired: 9 in, 1 out]
            n156 = property on="Test Slider" class="Slide (strict)"("Visible"=TRUE, "Scale.Maximum"=170.0 ("Scale.Range:Maximum")) -> ()  [unwired: 2 in, 2 out]
            n157 = local write "Test Slider"(w280) -> ()
            n158 = property on="Motor" class="Clust (strict)"("Visible"=w279) -> ()  [unwired: 2 in, 2 out]
            n159 = property on="Rev/Fwd" class="Clust (strict)"("Visible"=w279) -> ()  [unwired: 2 in, 2 out]
            n160 = property on="On/Off" class="Bool (strict)"("Visible"=w279) -> ()  [unwired: 2 in, 2 out]
            n161 = property on="Test Ring" class="Ring (strict)"("Visible"=w279) -> ()  [unwired: 2 in, 2 out]
          }
          frame "Relay", "Solenoid" {
            w282 = FALSE ("Visible")
            n162 = property on="Motor" class="Clust (strict)"("Visible"=w282) -> ()  [unwired: 2 in, 2 out]
            n163 = property on="Test Slider" class="Slide (strict)"("Visible"=w282) -> ()  [unwired: 2 in, 2 out]
            n164 = Search and Replace String(input string=w283, search string="/Value  **", replace string="/Direction") -> (result string=w289:string)  [unwired: 5 in, 3 out]
            n165 = property on="Test Ring" class="Ring (strict)"("Visible"=w282) -> ()  [unwired: 2 in, 2 out]
            n166 = call <vilib>:"NT Read String.vi"("Name"=w289) -> ("String"=w287:string)  [unwired: 9 in, 1 out]
            n167 = Equal?(x="Both directions", y=w287) -> (x = y?=w285:bool)
            n168 = Not(x=w285) -> (.not. x?=w286:bool)
            n169 = property on="Rev/Fwd" class="Clust (strict)"("Visible"=w285) -> ()  [unwired: 2 in, 2 out]
            n170 = property on="On/Off" class="Bool (strict)"("Visible"=w286, "Caption.Text"=w284) -> ()  [unwired: 2 in, 2 out]
          }
          frame "Compressor", "Digital Out" {
            w292 = FALSE ("Visible")
            # "Get direction and finish"
            n171 = property on="Motor" class="Clust (strict)"("Visible"=w292) -> ()  [unwired: 2 in, 2 out]
            n172 = property on="Test Slider" class="Slide (strict)"("Visible"=w292) -> ()  [unwired: 2 in, 2 out]
            n173 = property on="Test Ring" class="Ring (strict)"("Visible"=w292) -> ()  [unwired: 2 in, 2 out]
            n174 = property on="On/Off" class="Bool (strict)"("Visible"=TRUE, "Caption.Text"=w293) -> ()  [unwired: 2 in, 2 out]
            n175 = property on="Rev/Fwd" class="Clust (strict)"("Visible"=FALSE) -> ()  [unwired: 2 in, 2 out]
          }
          frame "Camera" {
            n176 = call <vilib>:"Get Last Path Segment.vi"("String in"=w300) -> ("String out"=w301:string)  [unwired: 10 in]
            n177 = property on="On/Off" class="Bool (strict)"("Visible"=FALSE) -> ()  [unwired: 2 in, 2 out]
            n178 = property on="Motor" class="Clust (strict)"("Visible"=FALSE) -> ()  [unwired: 2 in, 2 out]
            n179 = property on="Rev/Fwd" class="Clust (strict)"("Visible"=FALSE) -> ()  [unwired: 2 in, 2 out]
            n180 = case shown="\"White Balance  **\"" w301 {
              tunnel: w300 -> [w307 w316 w325 w334 w343 _ w349]
              tunnel: w299 -> [w305 w313 w322 w331 w340 _ _]
              frame "Size  **" {
                n181 = Index Array(array=w305) -> (element=w304:cluster{string[]})  [unwired: 1 in]
                n182 = call <vilib>:"NT Read String.vi"("Name"=w307) -> ("String"=w306:string)  [unwired: 9 in, 1 out]
                n183 = Unbundle(w304) -> (w302:string[])
                n184 = Match First String(2:w302, 3:w306) -> (0:w303:i32)  [unwired: 1 out]
                n185 = property on="Test Ring" class="Ring (strict)"("Value"=w303, "Strings []"=w302) -> ()  [unwired: 2 in, 2 out]
                n186 = property on="Test Ring" class="Ring (strict)"("Visible"=TRUE) -> ()  [unwired: 2 in, 2 out]
                n187 = property on="Test Slider" class="Slide (strict)"("Visible"=FALSE) -> ()  [unwired: 2 in, 2 out]
              }
              frame "White Balance  **" {
                n188 = Index Array(array=w313, index=1) -> (element=w314:cluster{string[]})
                n189 = call <vilib>:"NT Read String.vi"("Name"=w316) -> ("String"=w315:string)  [unwired: 9 in, 1 out]
                n190 = Unbundle(w314) -> (w311:string[])
                n191 = Match First String(2:w311, 3:w315) -> (0:w310:i32)  [unwired: 1 out]
                n192 = property on="Test Ring" class="Ring (strict)"("Value"=w310, "Strings []"=w311) -> ()  [unwired: 2 in, 2 out]
                n193 = property on="Test Ring" class="Ring (strict)"("Visible"=TRUE) -> ()  [unwired: 2 in, 2 out]
                n194 = property on="Test Slider" class="Slide (strict)"("Visible"=FALSE) -> ()  [unwired: 2 in, 2 out]
              }
              frame "Exposure  **" {
                n195 = Index Array(array=w322, index=2) -> (element=w323:cluster{string[]})
                n196 = call <vilib>:"NT Read String.vi"("Name"=w325) -> ("String"=w324:string)  [unwired: 9 in, 1 out]
                n197 = Unbundle(w323) -> (w319:string[])
                n198 = Match First String(2:w319, 3:w324) -> (0:w320:i32)  [unwired: 1 out]
                n199 = property on="Test Ring" class="Ring (strict)"("Value"=w320, "Strings []"=w319) -> ()  [unwired: 2 in, 2 out]
                n200 = property on="Test Ring" class="Ring (strict)"("Visible"=TRUE) -> ()  [unwired: 2 in, 2 out]
                n201 = property on="Test Slider" class="Slide (strict)"("Visible"=FALSE) -> ()  [unwired: 2 in, 2 out]
              }
              frame "Exposure Priority  **" {
                n202 = Index Array(array=w331, index=3) -> (element=w332:cluster{string[]})
                n203 = call <vilib>:"NT Read String.vi"("Name"=w334) -> ("String"=w333:string)  [unwired: 9 in, 1 out]
                n204 = Unbundle(w332) -> (w328:string[])
                n205 = Match First String(2:w328, 3:w333) -> (0:w329:i32)  [unwired: 1 out]
                n206 = property on="Test Ring" class="Ring (strict)"("Value"=w329, "Strings []"=w328) -> ()  [unwired: 2 in, 2 out]
                n207 = property on="Test Ring" class="Ring (strict)"("Visible"=TRUE) -> ()  [unwired: 2 in, 2 out]
                n208 = property on="Test Slider" class="Slide (strict)"("Visible"=FALSE) -> ()  [unwired: 2 in, 2 out]
              }
              frame "Color Enable  **" {
                n209 = Index Array(array=w340, index=4) -> (element=w341:cluster{string[]})
                n210 = call <vilib>:"NT Read String.vi"("Name"=w343) -> ("String"=w342:string)  [unwired: 9 in, 1 out]
                n211 = Unbundle(w341) -> (w337:string[])
                n212 = Match First String(2:w337, 3:w342) -> (0:w338:i32)  [unwired: 1 out]
                n213 = property on="Test Ring" class="Ring (strict)"("Value"=w338, "Strings []"=w337) -> ()  [unwired: 2 in, 2 out]
                n214 = property on="Test Ring" class="Ring (strict)"("Visible"=TRUE) -> ()  [unwired: 2 in, 2 out]
                n215 = property on="Test Slider" class="Slide (strict)"("Visible"=FALSE) -> ()  [unwired: 2 in, 2 out]
              }
              frame Default {
                n216 = property on="Test Ring" class="Ring (strict)"("Visible"=FALSE) -> ()  [unwired: 2 in, 2 out]
                n217 = property on="Test Slider" class="Slide (strict)"("Visible"=FALSE) -> ()  [unwired: 2 in, 2 out]
              }
              frame "Brightness  **", "Color Level  **", "Compression  **", "FPS  **", "Sharpness  **" {
                n218 = call <vilib>:"NT Read Number.vi"("Name"=w349) -> ("Numeric"=w348:dbl)  [unwired: 9 in, 1 out]
                n219 = local write "Test Slider"(w348) -> ()
                n220 = property on="Test Slider" class="Slide (strict)"("Visible"=TRUE, "Scale.Maximum"=100.0 ("Scale.Range:Maximum")) -> ()  [unwired: 2 in, 2 out]
                n221 = property on="Test Ring" class="Ring (strict)"("Visible"=FALSE) -> ()  [unwired: 2 in, 2 out]
              }
            }
          }
        }
        n222 = property on="Progress" class="Clust (strict)"("Visible"=FALSE) -> ()  [unwired: 2 in, 2 out]
      }
      event "Test Name": Mouse Enter {
        # "Populate the ring with the list of tests"
        n223 = event-data() -> ()  [unwired: 1 in, 1 out]
        n224 = call <vilib>:"NT Read String Array.vi"("Name"="/TestMode/TestList") -> ("String Array"=w357:string[])  [unwired: 9 in, 1 out]
        n225 = Build Array (concatenate)("Select the test to run...", w357) -> (w356:string[])
        n226 = property on="Test Name" class="Ring (strict)"("Strings []"=w356) -> ()  [unwired: 2 in, 2 out]
      }
      event "Test Name": Value Change {
        w359 = FALSE ("Visible")
        # "Tell the robot the test name to run"
        n227 = event-data() -> ("NewVal"=w363:u16)  [unwired: 1 in]
        n228 = property on="Test Name" class="Ring (strict)"() -> ("Strings []"=w364:string[])  [unwired: 2 in, 2 out]
        n229 = local write "Progress"(T5 {"Test Progress"=0, "Test Progress Text"=""} ("Progress")) -> ()
        n230 = Index Array(array=w364, index=w363) -> (element=w362:string)
        n231 = call <vilib>:"NT Write String.vi"("String"=w362, "Name"="/TestMode/TestName") -> ()  [unwired: 9 in, 1 out]
        n232 = property on="Progress" class="Clust (strict)"("Visible"=TRUE) -> ()  [unwired: 2 in, 2 out]
        n233 = property on="Motor" class="Clust (strict)"("Visible"=w359) -> ()  [unwired: 2 in, 2 out]
        n234 = property on="Test Slider" class="Slide (strict)"("Visible"=w359) -> ()  [unwired: 2 in, 2 out]
        n235 = property on="On/Off" class="Bool (strict)"("Visible"=w359) -> ()  [unwired: 2 in, 2 out]
        n236 = property on="Rev/Fwd" class="Clust (strict)"("Visible"=w359) -> ()  [unwired: 2 in, 2 out]
        n237 = property on="Test Ring" class="Ring (strict)"("Visible"=w359) -> ()  [unwired: 2 in, 2 out]
      }
      event "Command Selection": Value Change {
        # "Get the params and show in table"
        n238 = event-data() -> ("NewVal"=w369:i32)  [unwired: 1 in]
        n239 = property on="Command Selection" class="MCListbox (strict)"() -> ("ItemNames"=w367:string[][])  [unwired: 2 in, 2 out]
        n240 = call <vilib>:"WPI_DashboardUpdate Command Params.vi"("NewVal"=w369, "Commands"=w367, "Param Tbl"=w368) -> ()  [unwired: 8 in, 1 out]
      }
      event "Execute Command": Value Change {
        # "Started one, Unique ID holds\nresponse"
        n241 = event-data() -> ()  [unwired: 1 in, 1 out]
        n242 = property on="Command Selection" class="MCListbox (strict)"() -> ("ItemNames"=w380:string[][])  [unwired: 2 in, 2 out]
        n243 = Index Array(array=w380, index (row)="Command Selection", index (col)=0) -> (element=w378:string)
        n244 = call <vilib>:"Invoke Commands.vi"("Command Params"="Command Params", "Function Name"=w378) -> ("Params"=w374:u8, "Started"=w373:bool)  [unwired: 7 in, 1 out]
        n245 = Array Subset(array="Command Params", length (row)=w374) -> (w375:string[][])  [unwired: 3 in]
        n246 = Select(t="Executing" ("Cmd Status"), s=w373, f="" ("Cmd Status")) -> (s? t:f=→"Cmd Status":string)
      }
      event "Command Selection": Double Click {
        n247 = event-data() -> ("Row"=w388:i32)  [unwired: 1 in]
        n248 = property on="Command Selection" class="MCListbox (strict)"() -> ("ItemNames"=w391:string[][])  [unwired: 2 in, 2 out]
        n249 = local read "Command Params"() -> (w387:string[][])
        n250 = Index Array(array=w391, index (row)=w388, index (col)=0) -> (element=w389:string)
        n251 = call <vilib>:"Invoke Commands.vi"("Command Params"=w387, "Function Name"=w389) -> ("Params"=w386:u8, "Started"=w381:bool)  [unwired: 7 in, 1 out]
        n252 = Array Subset(array=w387, length (row)=w386) -> (w385:string[][])  [unwired: 3 in]
        n253 = Select(t="Executing" ("Cmd Status"), s=w381, f="" ("Cmd Status")) -> (s? t:f=w382:string)
        n254 = local write "Cmd Status"(w382) -> ()
      }
      event "CheckList": Double Click {
        # "Shift clears all"
        # "Update symbols on the listbox"
        n255 = event-data() -> ("PlatMods.Shift"=w393:bool, "Row"=w395:i32)  [unwired: 1 in]
        n256 = case shown="True" w393 {
          tunnel: w395 -> [w399 _]
          tunnel: 1 -> [w398 _]
          frame False {
            n257 = property on="CheckList" class="LstBox (strict)"() -> ("Item Symbols"=w397:i32[])  [unwired: 2 in, 2 out]
            n258 = Replace Array Subset(array=w397, new element=w398, index=w399) -> (w396:i32[])
            n259 = property on="CheckList" class="LstBox (strict)"("Item Symbols"=w396) -> ()  [unwired: 2 in, 2 out]
          }
          frame True {
            w400 = 0 ("Top Row")
            n260 = property on="CheckList" class="LstBox (strict)"() -> ("Number of Rows"=w402:u32)  [unwired: 2 in, 2 out]
            n261 = Initialize Array(0, w402) -> (w401:i32[])
            n262 = property on="CheckList" class="LstBox (strict)"("Top Row"=w400, "Value"=w400, "Item Symbols"=w401) -> ()  [unwired: 2 in, 2 out]
          }
        }
      }
      event "CheckList": Key Down {
        # "Update symbols on the listbox\nLeft and right keys check and uncheck"
        n263 = event-data() -> ("VKey"=w406:T15)  [unwired: 1 in]
        n264 = case shown="\"Left\", \"Right\"" w406 {
          selector: w406 -> [w411 _]
          tunnel: eventvkey."Left" ("VKey") -> [w409 _]
          frame "Left", "Right" {
            n265 = Equal?(x=w409, y=w411) -> (x = y?=w410:bool)
            n266 = Select(t=0, s=w410, f=1) -> (s? t:f=w412:i32)
            n267 = property on="CheckList" class="LstBox (strict)"() -> ("Item Symbols"=w415:i32[])  [unwired: 2 in, 2 out]
            n268 = Replace Array Subset(array=w415, new element=w412, index="CheckList") -> (w414:i32[])
            n269 = property on="CheckList" class="LstBox (strict)"("Item Symbols"=w414) -> ()  [unwired: 2 in, 2 out]
          }
          frame Default {
          }
        }
      }
      event "Motor.Enable": Value Change {
        # "When the test mode otor enable helper is set, update that\ntree row item's value"
        n270 = event-data() -> ("NewVal"=w421:bool)  [unwired: 1 in]
        n271 = Unbundle("Motor") -> ("Value"=w420:dbl)  [unwired: 1 out]
        n272 = Select(t=w420, s=w421, f=0.0) -> (s? t:f=w418:dbl)
        n273 = call <vilib>:"NT Write Number.vi"("Numeric"=w418, "Name"=w417) -> ()  [unwired: 9 in, 1 out]
      }
      event "Test Slider": Value Change {
        # "When the test mode slider helper is set, update that\ntree row item's value"
        n274 = event-data() -> ("NewVal"=w424:dbl)  [unwired: 1 in]
        n275 = call <vilib>:"NT Write Number.vi"("Numeric"=w424, "Name"=w425) -> ()  [unwired: 9 in, 1 out]
      }
      event "On/Off": Value Change {
        # "When the test mode on/off helper value is set, update that\ntree row item's value"
        n276 = event-data() -> ("NewVal"=w429:bool)  [unwired: 1 in]
        n277 = Boolean To (0,1)(Boolean=w429) -> (0, 1=w428:i16)
        n278 = call <vilib>:"NT Write Number.vi"("Numeric"=w428, "Name"=w427) -> ()  [unwired: 9 in, 1 out]
      }
      event "Rev/Fwd": Value Change {
        # "When the test mode helper value for relays is set, update that\ntree row item's value"
        n279 = event-data() -> ("NewVal.Forward"=w437:bool, "NewVal.Reverse"=w436:bool)  [unwired: 1 in]
        n280 = Boolean To (0,1)(Boolean=w437) -> (0, 1=w433:i16)
        n281 = Boolean To (0,1)(Boolean=w436) -> (0, 1=w435:i16)
        n282 = Negate(x=w435) -> (-x=w434:i16)
        n283 = Add(x=w433, y=w434) -> (x+y=w432:i16)
        n284 = call <vilib>:"NT Write Number.vi"("Numeric"=w432, "Name"=w431) -> ()  [unwired: 9 in, 1 out]
      }
      event "Test Ring": Value Change {
        # "When a test mode helper value is selected from the ring,\nset the tree item's variable to the string value"
        n285 = event-data() -> ("NewVal"=w441:u16)  [unwired: 1 in]
        n286 = property on="Test Ring" class="Ring (strict)"() -> ("Strings []"=w442:string[])  [unwired: 2 in, 2 out]
        n287 = Index Array(array=w442, index=w441) -> (element=w440:string)
        n288 = call <vilib>:"NT Write String.vi"("String"=w440, "Name"=w439) -> ()  [unwired: 9 in, 1 out]
      }
      event "Rec Mode": Value Change {
        # "Update globals for recording mode and path to read log from.\nClear when logging and let NetworkTables set path for vision to\nuse."
        n289 = event-data() -> ("NewVal"=w453:enum32{"Stop", "Record", "Playback"})  [unwired: 1 in]
        n290 = global write "WPI_DashboardLogging Global.vi" "Logging Filename"(path "") -> ()
        n291 = global write "WPI_DashboardLogging Global.vi" "Recording"(w453) -> ()
        n292 = case shown="\"Playback\"" w453 {
          tunnel: w452 -> [_ w455 w464]
          tunnel: [_ _ w463] -> w450
          tunnel: [_ _ w462] -> _
          tunnel: w448 -> [_ _ w460]
          tunnel: cluster{i32, i32} {-250, 170} -> [_ _ w459]
          tunnel: [_ _ T16 {"Image Size"=TRUE, "Image Type"=TRUE, "Pixel Value"=TRUE, "ROI Information"=TRUE, "Zoom Factor"=FALSE} ("Image Information Shown:All Elements")] -> w446
          tunnel: [_ _ TRUE ("Zoom Factor")] -> w445
          tunnel: w444 -> [_ _ w456]
          frame Default {
          }
          frame "Stop", "Record" {
            # "Place Window too"
            n293 = invoke class="VI" method="FP.Close"(reference=w455) -> (reference out=w454:refnum<vi>)  [unwired: 2 in, 2 out]
            n294 = invoke class="VI" method="Abort VI"(reference=w454) -> ()  [unwired: 2 in, 3 out]
          }
          frame "Playback" {
            n295 = call "Open Playback Panel.vi"("Offset"=w459, "DB VI Ref"=w460, "Playback in"=w464) -> ("Playback out"=w461:refnum<vi>)  [unwired: 8 in]
            n296 = register-events(w461, w456) -> (reference out=w463:refnum<event-registration>, error out=w462:errorcluster)  [unwired: 2 in]
          }
        }
        n297 = property on="Camera Image" class="ImageControl"("Image Information Shown"=w446, "Image Information Visible"=w445) -> ()  [unwired: 2 in, 2 out]
        n298 = call <vilib>:"WPI_DashboardNT Log FieldName Cache.vi"("Operation"=enum16{"Lookup/Add", "Index", "Clear"}."Clear") -> ()  [unwired: 8 in, 3 out]
      }
      event Panel Close {
        w466 = enum32{"Stop", "Record", "Playback"}."Stop" ("Rec Mode")
        # "Playback window has been closed, abort"
        n299 = event-data() -> ()  [unwired: 1 in, 4 out]
        n300 = local write "Rec Mode"(w466) -> ()
        n301 = global write "WPI_DashboardLogging Global.vi" "Recording"(w466) -> ()
      }
      event Panel Close {
        # "Abort playback window and ourself"
        n302 = event-data() -> ()  [unwired: 1 in, 4 out]
        n303 = invoke class="VI" method="FP.Close"(reference=w470) -> (reference out=w469:refnum<vi>)  [unwired: 2 in, 2 out]
        n304 = invoke class="VI" method="Abort VI"(reference=w469) -> (error out=w468:errorcluster)  [unwired: 2 in, 2 out]
        n305 = invoke class="VI" method="Abort VI"(error in=w468) -> ()  [unwired: 2 in, 3 out]
      }
      event User Event {
        n306 = event-data() -> ("IDs"=w477:cluster{"RPC field ID":u16, "Unique ID":u16}, "String"=w476:string)  [unwired: 1 in]
        n307 = Bundle("IDs"=w477, "String"=w476) -> (w475:T6)  [unwired: 1 in]
        n308 = call <vilib>:"Retrieve RPC Response.vi"("RPC Response"=w475) -> ("Output"=w473:string[][])  [unwired: 10 in]
        n309 = Build Array (concatenate)(w471, w473) -> (w472:string[][])
        n310 = local write "Command Params"(w472) -> ()
        n311 = local write "Cmd Status"("" ("Cmd Status")) -> ()
      }
      event "Tree": Double Click {
        n312 = event-data() -> ("PlatMods"=w481:T19, "Tag"=w480:string)  [unwired: 1 in]
        n313 = Unbundle(w481) -> ("Shift"=w479:bool)  [unwired: 4 out]
        n314 = Not(x=w479) -> (.not. x?=w478:bool)
        n315 = call <vilib>:"NT Update Persistence.vi"("Persistence"=w478, "Name"=w480) -> ()  [unwired: 9 in, 1 out]
      }
    }
  }
  n316 = while {
    tunnel: w58 -> [w484]
    i -> [w487]
    stop <- FALSE stop-if-true
    n317 = Wait (ms)(milliseconds to wait=u32 100) -> ()  [unwired: 1 out]
    n318 = case shown="\"Playback\"" "Rec Mode" {
      tunnel: w487 -> [_ _ w502]
      tunnel: [u32 2829099 ("Base Color") u32 11141120 ("Target Color") w491] -> w483
      frame "Stop", Default {
        # "Reset the color, extra updates don't cost much"
      }
      frame "Record" {
      }
      frame "Playback" {
        # "Playback"
        n319 = Quotient & Remainder(x=w502, y=u32 50 ("milliseconds to wait")) -> (x-y*floor(x/y)=w498:u32)  [unwired: 1 out]
        n320 = Divide(x=w498, y=u32 50 ("milliseconds to wait")) -> (x/y=w495:dbl)
        n321 = Multiply(x=6.283185307179586, y=w495) -> (x*y=w500:dbl)
        n322 = Sine(x=w500) -> (sin(x)=w499:dbl)
        n323 = Absolute Value(x=w499) -> (abs(x)=w492:dbl)
        n324 = call "Interpolate RGB Color.vi"("Proportion"=w492, "Target Color"=u32 30976, "Base Color"=u32 2829099) -> ("Result Color"=w491:u32)  [unwired: 8 in]
      }
    }
    n325 = property class="Pane"(reference=w484, "PaneColor"=w483) -> ()  [unwired: 1 in, 2 out]
  }
  n326 = local write "Dashboard Tab"(T2."Drive" ("Dashboard Tab")) -> ()
  n327 = property on="On/Off" class="Bool (strict)"("Visible"=w29) -> ()  [unwired: 2 in, 2 out]
  n328 = property on="Motor" class="Clust (strict)"("Visible"=w29) -> ()  [unwired: 2 in, 2 out]
  n329 = property on="Progress" class="Clust (strict)"("Visible"=w29) -> ()  [unwired: 2 in, 2 out]
  n330 = property on="Test Ring" class="Ring (strict)"("Visible"=w29) -> ()  [unwired: 2 in, 2 out]
  n331 = property on="Rev/Fwd" class="Clust (strict)"("Visible"=w29) -> ()  [unwired: 2 in, 2 out]
  n332 = while {
    tunnel: u16 1741 ("timeout ms (25000)") -> [w504]
    stop <- FALSE stop-if-true
    n333 = TCP Create Listener(10:w504) -> (0:w503:errorcluster, 3:w505:refnum<k5>)  [unwired: 4 in, 1 out]
    n334 = case shown="No Error" w503 {
      selector: w503 -> [w507 _]
      tunnel: w505 -> [w508 _]
      frame No Error {
        n335 = while {
          tunnel: w508 -> [w511]
          tunnel: w507 -> [w510]
          stop <- FALSE stop-if-true
          n336 = TCP Wait On Listener(8:w510, 11:w511) -> (0:w512:errorcluster, 4:w513:refnum<k5>)  [unwired: 2 in, 3 out]
          n337 = local write "TCP"(w513) -> ()
          n338 = case shown="No Error" w512 {
            frame No Error {
            }
            frame Error {
              n339 = Wait (ms)(milliseconds to wait=u32 1000) -> ()  [unwired: 1 out]
            }
          }
        }
      }
      frame Error {
        n340 = Wait (ms)(milliseconds to wait=u32 1000) -> ()  [unwired: 1 out]
      }
    }
  }
  n341 = local write "Command Selection"(u16 0 ("milliseconds to wait")) -> ()
  n342 = local write "Command Params"(string[][] [] ("Command Params")) -> ()
  n343 = global write "WPI_DashboardLogging Global.vi" "Recording"(w52) -> ()
  n344 = local write "Rec Mode"(w52) -> ()
